vi "Instantiate.vi"(1 "vi ref":refnum<vi>) -> (0 "vi ref":refnum<vi>)   [LabVIEW 2020, in "BasicChannelWireForkable.lvlib"]
doc: "This is the VI that gets automatically inserted at the root of a Channel Wire.\n\nChannel Wires in fact DO follow dataflow paradigms with the caveat that the LabVIEW compiler treats all <b>indicators</b> (structure/subVI OUTPUTS) as <b>controls</b> (structure/subVI INPUTS). This is why Channel Wires can't flow through structures, any terminal needs to flow INTO the structure/node which would mean inside the structure, two inputs get connected which isn't allowed.\n\nThis Initialization.vi is automatically inserted by the compiler into the \"root\" segment of a Channel Wire and then the reference to the internal handling VI flows from there."
uses:
  BasicChannelWireForkable.lvlib
  ))Channel.vi
  Operation.ctl
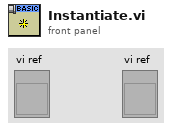
[diagram p1: front panel]
types:
  T1 = typedef "BasicChannelWireForkable.lvlib/Operation.ctl" = enum16{"Init", "Get Core", "Close"}
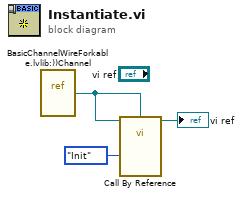
[diagram p0: block diagram]
diagram:
  n1 = vi-ref "BasicChannelWireForkable.lvlib:))Channel.vi"() -> (w2:refnum<vi>)
  n2 = call-by-ref "?"(reference=w2, "VI Ref In"=w2, "Operation"=Operation."Init") -> (reference out=→"vi ref":refnum<vi>)  [unwired: 13 in, 3 out]
